vi "Facade.vi"(0 "Data In":T4, 2 "Display State In":T2, 3 "Container State":T3) -> (6 "Data Out":T4, 7 "Display State Out":T2, 8 "Action":T1)   [LabVIEW 2014, in "Xgraph.xctl"]
uses:
  Xgraph.xctl
  Data.ctl
  <vilib>/_xctls/Container State.ctl
  State.ctl
  <vilib>/_xctls/Action.ctl
  <vilib>/_xctls/XControlSupport.lvlib
panel:
  in  "录波?":bool caption="录波"
  out "波形文件大小":string
  out "已录波":string
  out "录波开始时间":string
  in  "模式选择":u16(ring) items=["示波模式", "录波模式", "XY图模式"]
  out "XY Graph":cluster{"Y":dbl[], "Y":dbl[]}[](graph)
  in  "Choose 2":u16(ring) items=["Estlalpha", "AlphaErr", "speed", "iq", "id"]
  in  "Choose 1":u16(ring) items=["Estlalpha", "AlphaErr", "speed", "iq", "id"]
  in  "时频域转换 2":bool
  out "Graph 2":dbl[](graph)
  in  "时频域转换 1":bool
  out "Graph 1":dbl[](graph)
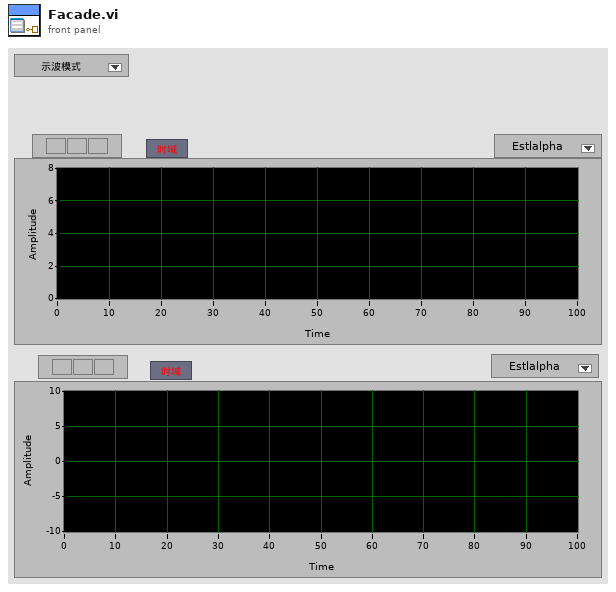
[diagram p1: front panel]
types:
  T1 = typedef "XControlSupport.lvlib/Action.ctl" = cluster{"Data Changed?":bool, "State Changed?":bool, "Action Name":string}
  T2 = typedef "Xgraph.xctl/State.ctl" = cluster{"时频1":refnum<vi>, "时频2":refnum<vi>, "Cho1":refnum<vi>, "Cho2":refnum<vi>}
  T3 = typedef "XControlSupport.lvlib/Container State.ctl" = cluster{"Indicator?":bool, "Run Mode?":bool, " Refnum":refnum<vi>}
  T4 = typedef "Xgraph.xctl/Data.ctl" = cluster{"Data1":dbl[], "Data2":dbl[]}
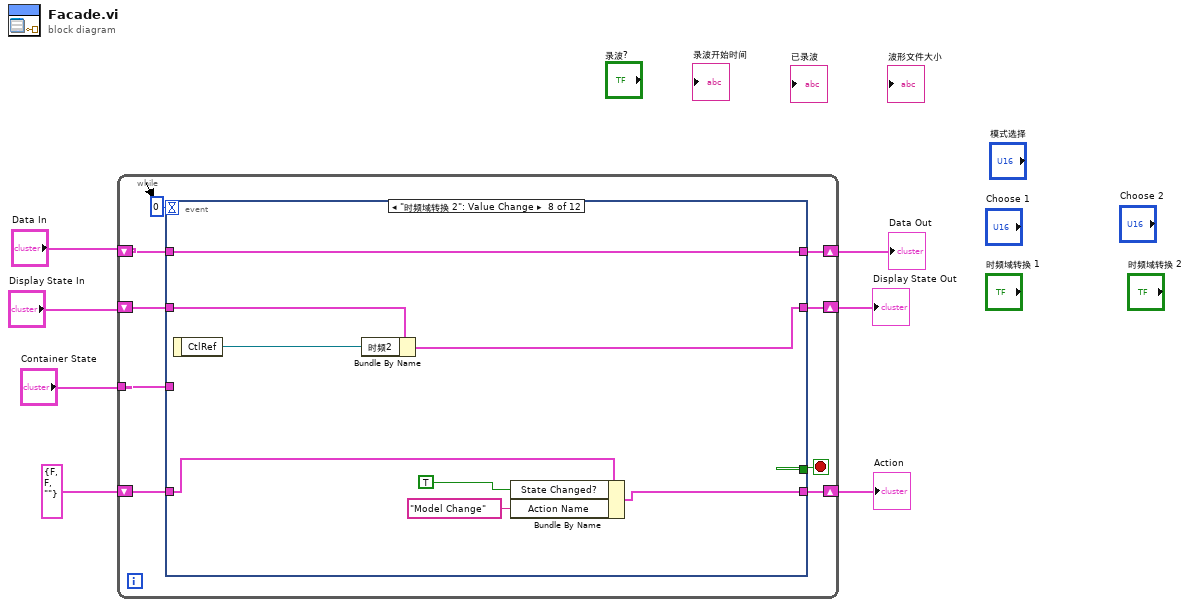
[diagram p0: block diagram]
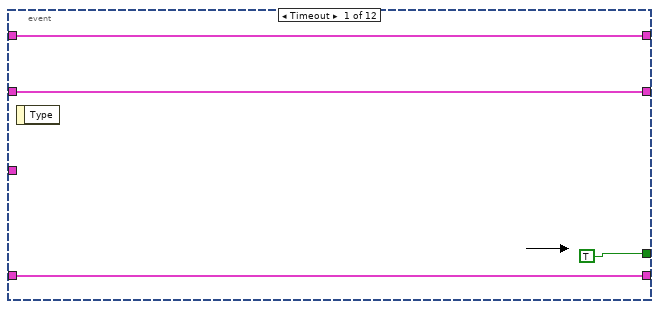
[diagram p2: hidden frame]
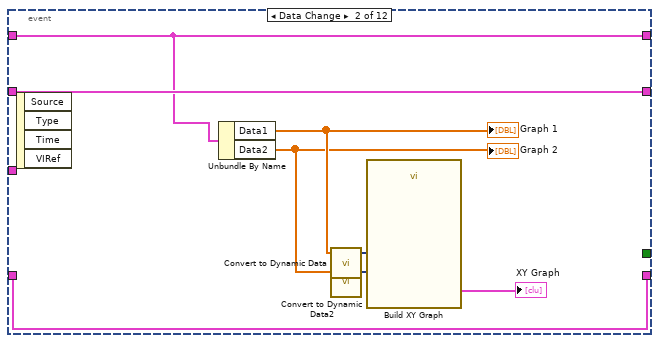
[diagram p3: hidden frame]
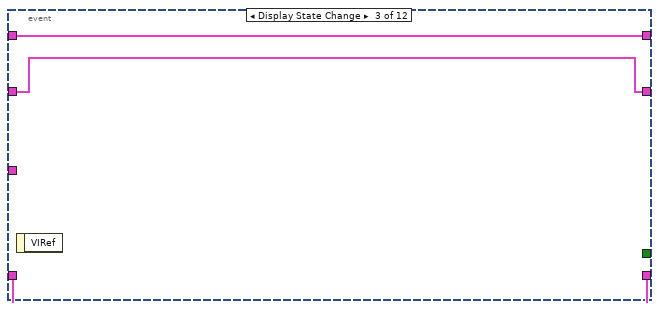
[diagram p4: hidden frame]
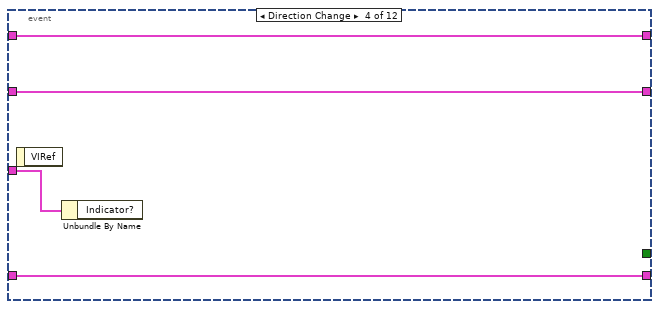
[diagram p5: hidden frame]
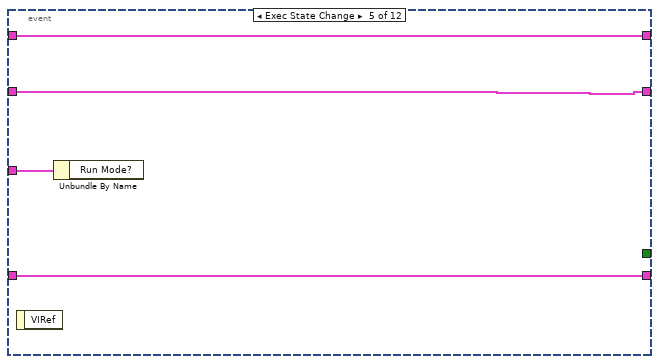
[diagram p6: hidden frame]
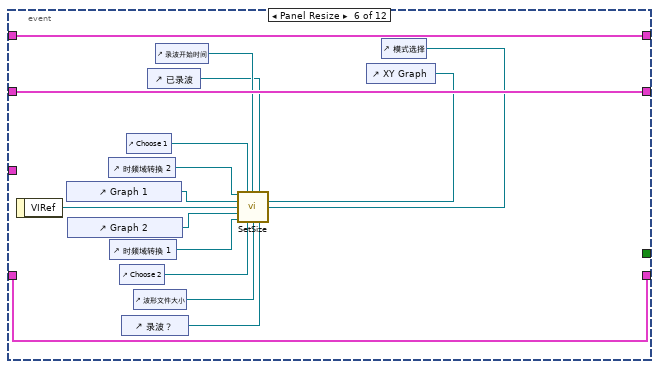
[diagram p7: hidden frame]
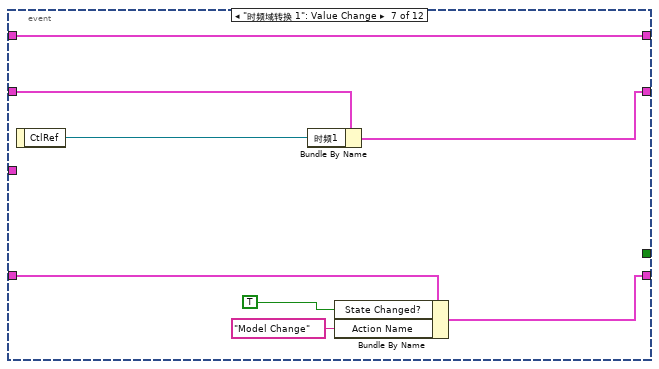
[diagram p8: hidden frame]
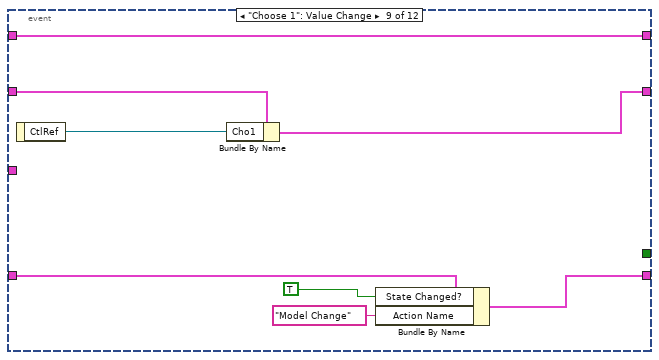
[diagram p9: hidden frame]
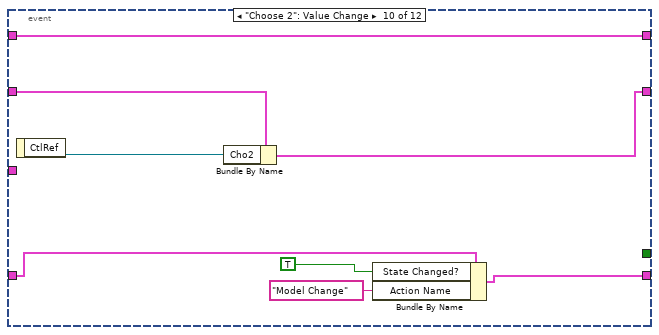
[diagram p10: hidden frame]
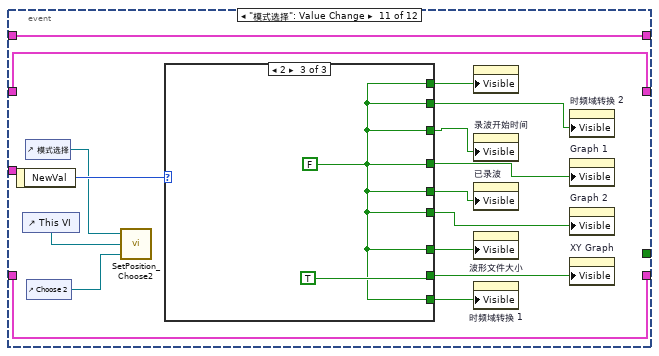
[diagram p11: hidden frame]
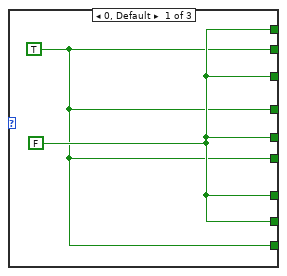
[diagram p12: hidden frame]
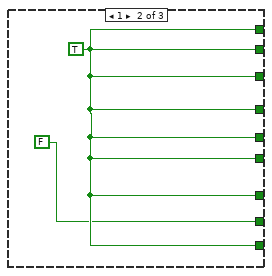
[diagram p13: hidden frame]
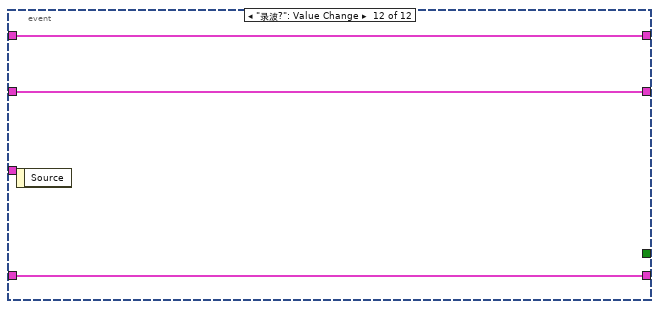
[diagram p14: hidden frame]
diagram:
  n1 = while {
    shift-right: [w15] -> w1
    shift-left: "Display State In" -> [w16]
    tunnel: "Container State" -> [w12]
    shift-right: [w10] -> w7
    shift-left: "Data In" -> [w11]
    shift-right: [w8] -> w4
    shift-left: T1 {"Data Changed?"=FALSE, "State Changed?"=FALSE, "Action Name"=""} ("Action") -> [w9]
    stop <- w14 stop-if-true
    n2 = event shown="[7] \"时频域转换 2\": Value Change" {
      selector: _ -> [_ _ _ _ _ _ _ _ _ _ _ _]
      dyn-events: _ -> [_ _ _ _ _ _ _ _ _ _ _ _]
      timeout: 0 -> [_ _ _ _ _ _ _ _ _ _ _ _]
      tunnel: w16 -> [w17 w27 w29 w34 w36 w53 w57 w64 w76 w84 w103 w112]
      tunnel: [w17 w27 w29 w34 w36 w53 w62 w68 w75 w82 w103 w112] -> w15
      tunnel: [TRUE _ _ _ _ _ _ _ _ _ _ _] -> w14
      tunnel: w12 -> [_ _ _ w35 w39 _ _ _ _ _ _ _]
      tunnel: w11 -> [w18 w26 w31 w33 w38 w55 w63 w71 w79 w87 w102 w111]
      tunnel: [w18 w26 w31 w33 w38 w55 w63 w71 w79 w87 w102 w111] -> w10
      tunnel: [w19 w28 w30 w32 w37 w54 w58 w66 w74 w80 w101 w110] -> w8
      tunnel: w9 -> [w19 w28 w30 w32 w37 w54 w61 w65 w73 w81 w101 w110]
      event Timeout {
        n3 = event-data() -> ()  [unwired: 1 in, 1 out]
      }
      event Data Change {
        n4 = event-data() -> ()  [unwired: 1 in, 4 out]
        n5 = Unbundle By Name(w26) -> ("Data1"=w24:dbl[], "Data2"=w22:dbl[])
        "Graph 1" <- w24
        "Graph 2" <- w22
        n6 = call "Convert to Dynamic Data"("Array"=w24) -> ("Dynamic Data Type"=w23:dynamicdata)  [unwired: 3 in]
        n7 = call "Convert to Dynamic Data2"("Array"=w22) -> ("Dynamic Data Type"=w21:dynamicdata)  [unwired: 3 in]
        n8 = call "Build XY Graph"("Y Input"=w21, "X Input"=w23) -> ("XY Graph"=→"XY Graph":cluster{"X":dbl[], "Y":dbl[]}[])  [unwired: 8 in, 1 out]
      }
      event Display State Change {
        n9 = event-data() -> ()  [unwired: 1 in, 1 out]
      }
      event Direction Change {
        n10 = event-data() -> ()  [unwired: 1 in, 1 out]
        n11 = Unbundle By Name(w35) -> ()  [unwired: 1 out]
      }
      event Exec State Change {
        n12 = event-data() -> ()  [unwired: 1 in, 1 out]
        n13 = Unbundle By Name(w39) -> ()  [unwired: 1 out]
      }
      event Panel Resize {
        n14 = event-data() -> ("VIRef"=w52:refnum<vi>)  [unwired: 1 in]
        n15 = control-ref of="Graph 1"() -> (w51:refnum<vi>)
        n16 = control-ref of="Graph 2"() -> (w50:refnum<vi>)
        n17 = control-ref of="时频域转换 2"() -> (w49:refnum<vi>)
        n18 = control-ref of="时频域转换 1"() -> (w48:refnum<vi>)
        n19 = control-ref of="Choose 2"() -> (w46:refnum<vi>)
        n20 = control-ref of="录波？"() -> (w40:refnum<vi>)
        n21 = control-ref of="Choose 1"() -> (w47:refnum<vi>)
        n22 = control-ref of="波形文件大小"() -> (w41:refnum<vi>)
        n23 = control-ref of="已录波"() -> (w42:refnum<vi>)
        n24 = control-ref of="录波开始时间"() -> (w43:refnum<vi>)
        n25 = control-ref of="XY Graph"() -> (w44:refnum<vi>)
        n26 = control-ref of="模式选择"() -> (w45:refnum<vi>)
        n27 = call "SetSize.vi"("时频域1"=w49, "Choose1"=w47, "录波开始时间"=w43, "已录波"=w42, "Graph1"=w51, "XYGraph"=w44, "FcdVI Refnum"=w52, "Mode"=w45, "Graph2"=w50, "时频域2"=w48, "Choose2"=w46, "录波文件大小"=w41, "录波？"=w40) -> ()  [unwired: 3 in]
      }
      event "时频域转换 1": Value Change {
        n28 = event-data() -> ("CtlRef"=w56:refnum<vi>)  [unwired: 1 in]
        n29 = Bundle By Name(cluster=w57, "时频1"=w56) -> (w62:T2)
        n30 = Bundle By Name(cluster=w61, "State Changed?"=TRUE, "Action Name"="Model Change") -> (w58:T1)
      }
      event "时频域转换 2": Value Change {
        n31 = event-data() -> ("CtlRef"=w67:refnum<vi>)  [unwired: 1 in]
        n32 = Bundle By Name(cluster=w64, "时频2"=w67) -> (w68:T2)
        n33 = Bundle By Name(cluster=w65, "State Changed?"=TRUE, "Action Name"="Model Change") -> (w66:T1)
      }
      event "Choose 1": Value Change {
        n34 = event-data() -> ("CtlRef"=w72:refnum<vi>)  [unwired: 1 in]
        n35 = Bundle By Name(cluster=w76, "Cho1"=w72) -> (w75:T2)
        n36 = Bundle By Name(cluster=w73, "State Changed?"=TRUE, "Action Name"="Model Change") -> (w74:T1)
      }
      event "Choose 2": Value Change {
        n37 = event-data() -> ("CtlRef"=w83:refnum<vi>)  [unwired: 1 in]
        n38 = Bundle By Name(cluster=w84, "Cho2"=w83) -> (w82:T2)
        n39 = Bundle By Name(cluster=w81, "State Changed?"=TRUE, "Action Name"="Model Change") -> (w80:T1)
      }
      event "模式选择": Value Change {
        n40 = event-data() -> ("NewVal"=w100:u16)  [unwired: 1 in]
        n41 = control-ref of="This VI"() -> (w88:refnum<vi>)
        n42 = control-ref of="模式选择"() -> (w90:refnum<vi>)
        n43 = control-ref of="Choose 2"() -> (w89:refnum<vi>)
        n44 = call "SetPosition_Choose2.vi"("Choose2"=w89, "FcdVI Refnum"=w88, "Mode"=w90) -> ()
        n45 = case shown="2" w100 {
          tunnel: [w105 w107 w108] -> w99
          tunnel: [w104 w107 w108] -> w98
          tunnel: [w105 w107 w108] -> w97
          tunnel: [w104 w107 w108] -> w96
          tunnel: [w105 w107 w108] -> w95
          tunnel: [w104 w107 w108] -> w94
          tunnel: [w105 w107 w108] -> w93
          tunnel: [w105 FALSE TRUE] -> w92
          tunnel: [w104 w107 w108] -> w91
          frame 0, Default {
            w105 = FALSE
            w104 = TRUE
          }
          frame 1 {
            w107 = TRUE
          }
          frame 2 {
            w108 = FALSE
          }
        }
        n46 = property on="录波?" class="Bool (strict)"("Visible"=w99) -> ()  [unwired: 2 in, 2 out]
        n47 = property on="录波开始时间" class="Str"("Visible"=w97) -> ()  [unwired: 2 in, 2 out]
        n48 = property on="已录波" class="Str"("Visible"=w95) -> ()  [unwired: 2 in, 2 out]
        n49 = property on="波形文件大小" class="Str"("Visible"=w93) -> ()  [unwired: 2 in, 2 out]
        n50 = property on="时频域转换 1" class="Bool (strict)"("Visible"=w91) -> ()  [unwired: 2 in, 2 out]
        n51 = property on="时频域转换 2" class="Bool (strict)"("Visible"=w98) -> ()  [unwired: 2 in, 2 out]
        n52 = property on="Graph 1" class="WFGraph (strict)"("Visible"=w96) -> ()  [unwired: 2 in, 2 out]
        n53 = property on="Graph 2" class="WFGraph (strict)"("Visible"=w94) -> ()  [unwired: 2 in, 2 out]
        n54 = property on="XY Graph" class="XYGraph (strict)"("Visible"=w92) -> ()  [unwired: 2 in, 2 out]
      }
      event "录波?": Value Change {
        n55 = event-data() -> ()  [unwired: 1 in, 1 out]
      }
    }
  }
  "Display State Out" <- w1
  "Data Out" <- w7
  "Action" <- w4
